vi "Configure Stop Arming.vi"(5 "External Stop Arm Delay (0.001 s)":dbl=0.001, 7 "Stop Arming Type (0:Immediate)":i32(ring) items=["Immediate", "External"], 8 "error in (no error)":errorcluster, 9 "External Stop Arm Slope (0:Positive)":i32(ring) items=["Positive", "Negative"], 10 "External Stop Arm Source (1:Channel 1)":i32(ring)=1 items=["Channel 1"=1, "Channel 2"=2], 11 "VISA resource name":refnum<visa-resource-name>) -> (0 "error out":errorcluster, 3 "VISA resource name out":refnum<visa-resource-name>)   [LabVIEW 2020, in "Template - Counter.lvlib"]
doc: "Configures the parameters required for stop arming. This VI should be called after the <b>Configure Measurement</b> VI."
uses:
  <instrlib>/_Template - Counter/Template - Counter.lvlib
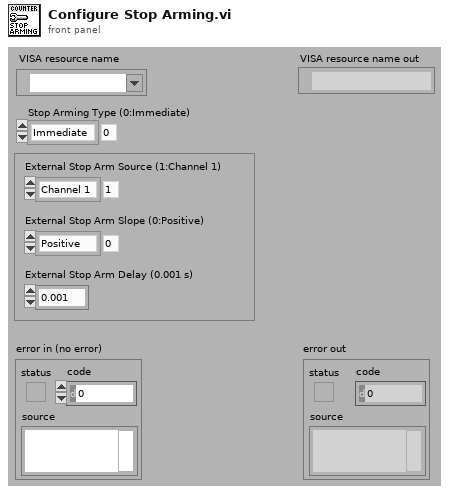
[diagram p1: front panel]
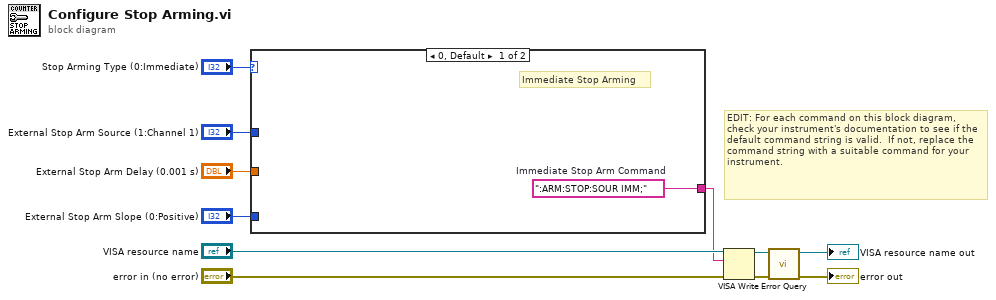
[diagram p0: block diagram]
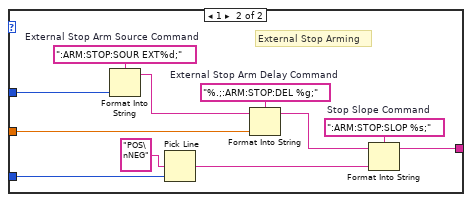
[diagram p2: hidden frame]
diagram:
  # "EDIT: For each command on this block diagram, check your instrument's documentation to see if the default command string is valid.  If not, replace the command string with a suitable command for your instrument."
  n1 = case shown="0, Default" "Stop Arming Type (0:Immediate)" {
    tunnel: [w12 w13] -> w5
    tunnel: "External Stop Arm Slope (0:Positive)" -> [_ w20]
    tunnel: "External Stop Arm Source (1:Channel 1)" -> [_ w18]
    tunnel: "External Stop Arm Delay (0.001 s)" -> [_ w15]
    frame 0, Default {
      w12 = ":ARM:STOP:SOUR IMM;"  # Immediate Stop Arm Command
      # "Immediate Stop Arming"
    }
    frame 1 {
      w17 = "%.;:ARM:STOP:DEL %g;"  # External Stop Arm Delay Command
      w21 = ":ARM:STOP:SLOP %s;"  # Stop Slope Command
      w19 = ":ARM:STOP:SOUR EXT%d;"  # External Stop Arm Source Command
      # "External Stop Arming"
      n2 = Format Into String(format string=w19, w18) -> (resulting string=w16:string)  [unwired: 2 in, 1 out]
      n3 = Pick Line(multi-line string="POS\nNEG", line index=w20) -> (output string=w22:string)  [unwired: 1 in]
      n4 = Format Into String(format string=w17, initial string=w16, w15) -> (resulting string=w14:string)  [unwired: 1 in, 1 out]
      n5 = Format Into String(format string=w21, initial string=w14, w22) -> (resulting string=w13:string)  [unwired: 1 in, 1 out]
    }
  }
  n6 = VISA Write(VISA resource name="VISA resource name", write buffer=w5, error in (no error)="error in (no error)") -> (VISA resource name out=w11:refnum<visa-resource-name>, error out=w10:errorcluster)  [unwired: 1 out]
  n7 = call <instrlib>:"Error Query.vi"("error in (no error)"=w10, "VISA resource name"=w11) -> ("error out"=→"error out":errorcluster, "VISA resource name out"=→"VISA resource name out":refnum<visa-resource-name>)  [unwired: 6 in, 2 out]
